vi "MovementDirections.vi"(9 "Key input":T1, 10 "Level input":u32[][](array[colorbox]), 11 "Location input":cluster{"Y":i32, "X":i32}[](array[cluster])=[{"Y"=12, "X"=8}, {"Y"=12, "X"=7}, {"Y"=12, "X"=6}, {"Y"=12, "X"=5}]) -> (1 "Key output":T1, 2 "Level output":u32[][](array[colorbox]), 3 "Location output":cluster{"Y":i32, "X":i32}[](array[cluster])=[{"Y"=12, "X"=8}, {"Y"=12, "X"=7}, {"Y"=12, "X"=6}, {"Y"=12, "X"=5}])   [LabVIEW 2021]
uses:
  TypeDef/KeyDown.ctl
  GlobalVariables/Board_Colors.vi
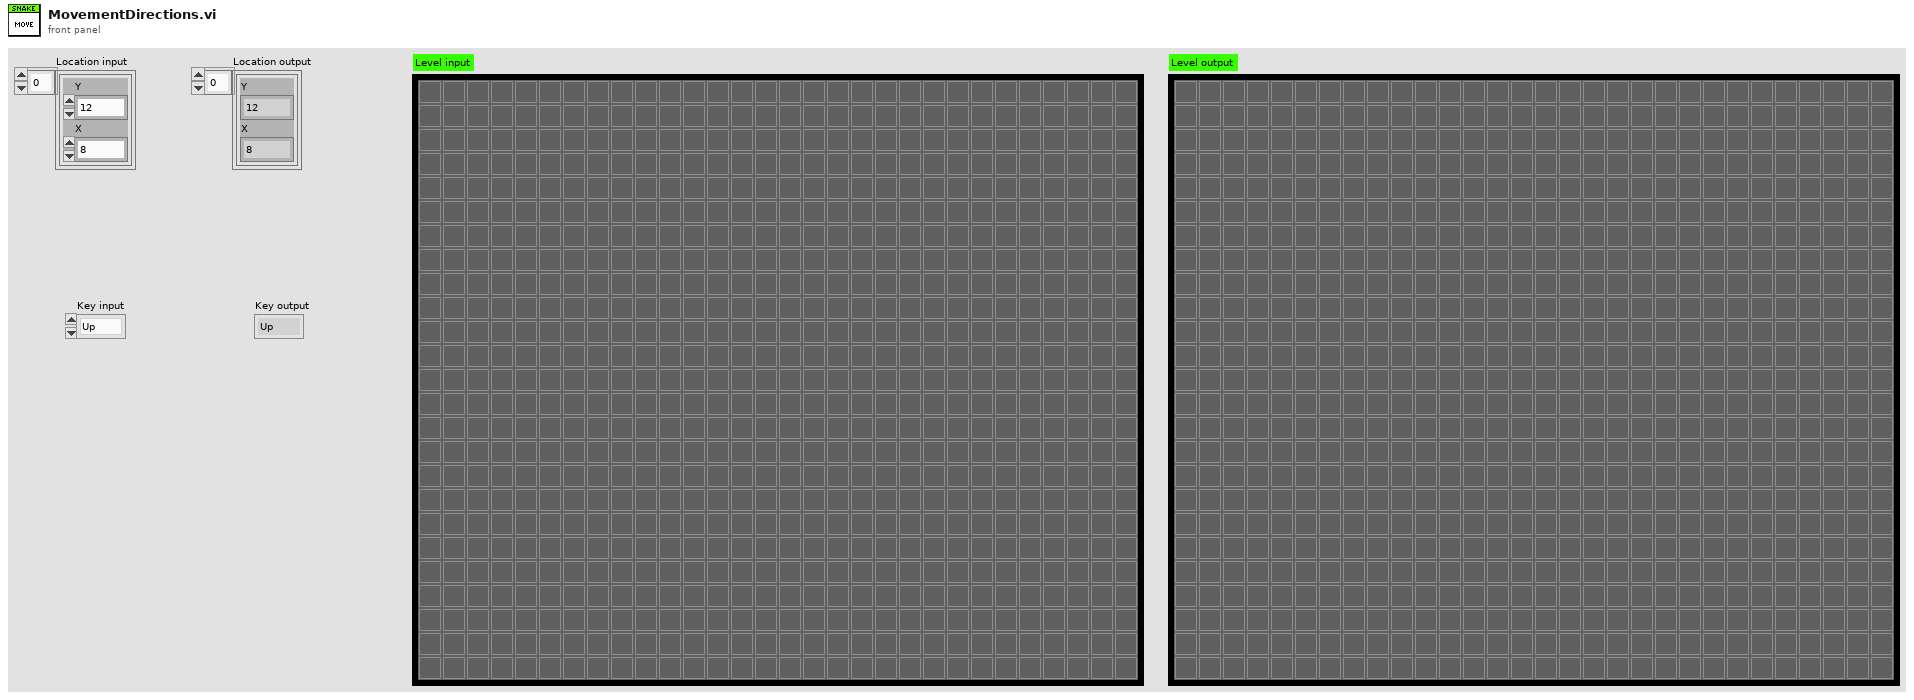
[diagram p1: front panel]
types:
  T1 = typedef "KeyDown.ctl" = enum16{"Up", "Down", "Left", "Right"}
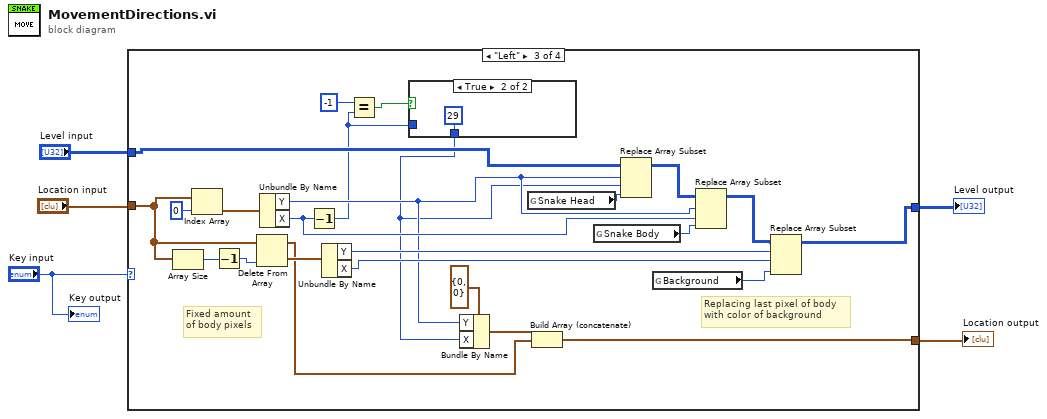
[diagram p0: block diagram]
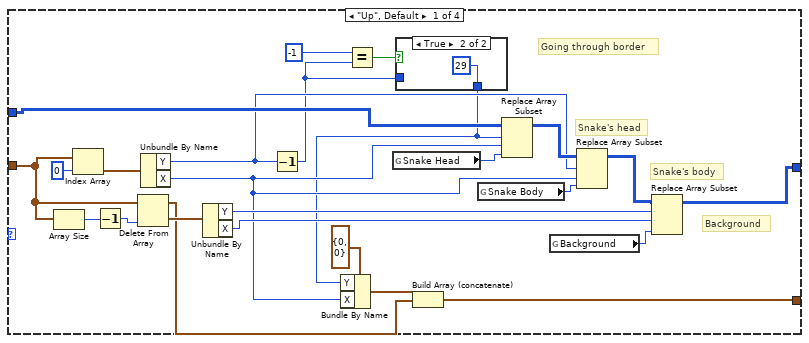
[diagram p2: hidden frame]
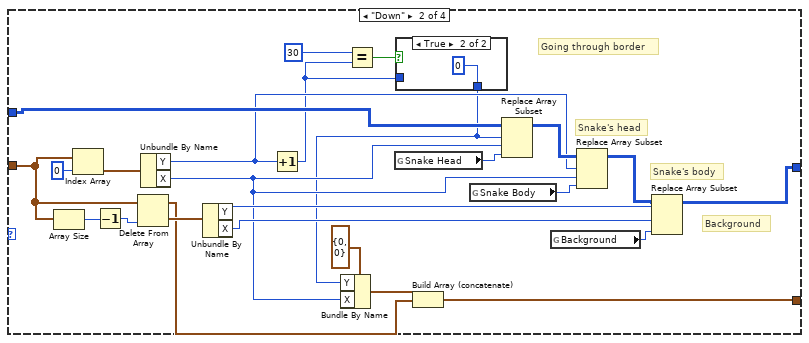
[diagram p4: hidden frame]
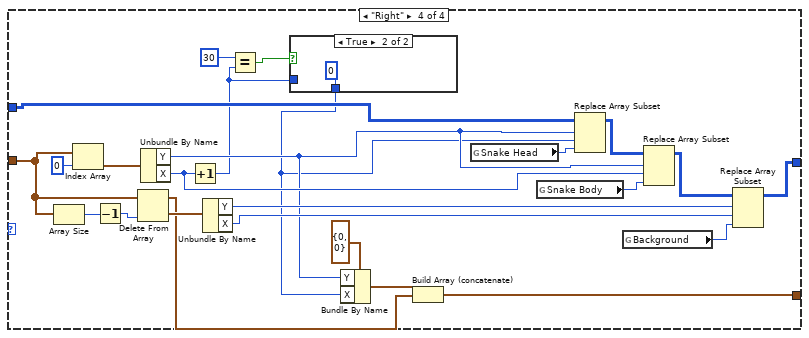
[diagram p7: hidden frame]
diagram:
  n1 = case shown="\"Left\"" "Key input" {
    tunnel: "Level input" -> [w27 w54 w81 w108]
    tunnel: [w22 w49 w75 w102] -> w3
    tunnel: "Location input" -> [w19 w46 w71 w98]
    tunnel: [w15 w42 w67 w94] -> w1
    frame "Up", Default {
      # "Background"
      # "Snake's body"
      # "Snake's head"
      # "Going through border"
      n2 = Array Size(array=w19) -> (size(s)=w28:i32)
      n3 = Index Array(array=w19, index=0) -> (element=w29:cluster{"Y":i32, "X":i32})
      n4 = Decrement(x=w28) -> (x-1=w18:i32)
      n5 = Delete From Array(array=w19, index=w18) -> (deleted portion=w17:cluster{"Y":i32, "X":i32}, array with subset deleted=w16:cluster{"Y":i32, "X":i32}[])  [unwired: 1 in]
      n6 = Unbundle By Name(w29) -> ("Y"=w13:i32, "X"=w14:i32)
      n7 = Unbundle By Name(w17) -> ("Y"=w24:i32, "X"=w23:i32)
      n8 = Decrement(x=w13) -> (x-1=w10:i32)
      n9 = Equal?(x=-1, y=w10) -> (x = y?=w12:bool)
      n10 = global read "Board_Colors.vi" "Snake Head"() -> (w6:u32)
      n11 = case shown="True" w12 {
        tunnel: [w31 29] -> w9
        tunnel: w10 -> [w31 _]
        frame False {
        }
        frame True {
        }
      }
      n12 = Bundle By Name(cluster=cluster{"Y":i32, "X":i32} {"Y"=0, "X"=0} ("input cluster"), "Y"=w9, "X"=w14) -> (w20:cluster{"Y":i32, "X":i32})
      n13 = Build Array (concatenate)(w20, w16) -> (w15:cluster{"Y":i32, "X":i32}[])
      n14 = global read "Board_Colors.vi" "Snake Body"() -> (w7:u32)
      n15 = Replace Array Subset(array=w27, new element=w6, index (row)=w9, index (col)=w14) -> (w26:u32[][])
      n16 = global read "Board_Colors.vi" "Background"() -> (w8:u32)
      n17 = Replace Array Subset(array=w26, new element=w7, index (row)=w13, index (col)=w14) -> (w25:u32[][])
      n18 = Replace Array Subset(array=w25, new element=w8, index (row)=w24, index (col)=w23) -> (w22:u32[][])
    }
    frame "Down" {
      # "Background"
      # "Snake's body"
      # "Snake's head"
      # "Going through border"
      n19 = Array Size(array=w46) -> (size(s)=w55:i32)
      n20 = Index Array(array=w46, index=0) -> (element=w56:cluster{"Y":i32, "X":i32})
      n21 = Decrement(x=w55) -> (x-1=w45:i32)
      n22 = Delete From Array(array=w46, index=w45) -> (deleted portion=w44:cluster{"Y":i32, "X":i32}, array with subset deleted=w43:cluster{"Y":i32, "X":i32}[])  [unwired: 1 in]
      n23 = Unbundle By Name(w56) -> ("Y"=w40:i32, "X"=w41:i32)
      n24 = Unbundle By Name(w44) -> ("Y"=w51:i32, "X"=w50:i32)
      n25 = Increment(x=w40) -> (x+1=w37:i32)
      n26 = Equal?(x=30, y=w37) -> (x = y?=w39:bool)
      n27 = global read "Board_Colors.vi" "Snake Head"() -> (w33:u32)
      n28 = case shown="True" w39 {
        tunnel: [w58 0] -> w36
        tunnel: w37 -> [w58 _]
        frame False {
        }
        frame True {
        }
      }
      n29 = Bundle By Name(cluster=cluster{"Y":i32, "X":i32} {"Y"=0, "X"=0} ("input cluster"), "Y"=w36, "X"=w41) -> (w47:cluster{"Y":i32, "X":i32})
      n30 = Build Array (concatenate)(w47, w43) -> (w42:cluster{"Y":i32, "X":i32}[])
      n31 = global read "Board_Colors.vi" "Snake Body"() -> (w34:u32)
      n32 = Replace Array Subset(array=w54, new element=w33, index (row)=w36, index (col)=w41) -> (w53:u32[][])
      n33 = global read "Board_Colors.vi" "Background"() -> (w35:u32)
      n34 = Replace Array Subset(array=w53, new element=w34, index (row)=w40, index (col)=w41) -> (w52:u32[][])
      n35 = Replace Array Subset(array=w52, new element=w35, index (row)=w51, index (col)=w50) -> (w49:u32[][])
    }
    frame "Left" {
      # "Fixed amount\nof body pixels"
      # "Replacing last pixel of body\nwith color of background"
      n36 = Array Size(array=w71) -> (size(s)=w82:i32)
      n37 = Index Array(array=w71, index=0) -> (element=w83:cluster{"Y":i32, "X":i32})
      n38 = Decrement(x=w82) -> (x-1=w70:i32)
      n39 = Delete From Array(array=w71, index=w70) -> (deleted portion=w69:cluster{"Y":i32, "X":i32}, array with subset deleted=w68:cluster{"Y":i32, "X":i32}[])  [unwired: 1 in]
      n40 = Unbundle By Name(w83) -> ("Y"=w74:i32, "X"=w76:i32)
      n41 = Decrement(x=w76) -> (x-1=w63:i32)
      n42 = Unbundle By Name(w69) -> ("Y"=w78:i32, "X"=w77:i32)
      n43 = Equal?(x=-1, y=w63) -> (x = y?=w65:bool)
      n44 = case shown="True" w65 {
        tunnel: [w85 29] -> w64
        tunnel: w63 -> [w85 _]
        frame False {
        }
        frame True {
        }
      }
      n45 = Bundle By Name(cluster=cluster{"Y":i32, "X":i32} {"Y"=0, "X"=0} ("input cluster"), "Y"=w74, "X"=w64) -> (w72:cluster{"Y":i32, "X":i32})
      n46 = global read "Board_Colors.vi" "Snake Head"() -> (w61:u32)
      n47 = Build Array (concatenate)(w72, w68) -> (w67:cluster{"Y":i32, "X":i32}[])
      n48 = global read "Board_Colors.vi" "Snake Body"() -> (w60:u32)
      n49 = Replace Array Subset(array=w81, new element=w61, index (row)=w74, index (col)=w64) -> (w80:u32[][])
      n50 = global read "Board_Colors.vi" "Background"() -> (w62:u32)
      n51 = Replace Array Subset(array=w80, new element=w60, index (row)=w74, index (col)=w76) -> (w79:u32[][])
      n52 = Replace Array Subset(array=w79, new element=w62, index (row)=w78, index (col)=w77) -> (w75:u32[][])
    }
    frame "Right" {
      n53 = Array Size(array=w98) -> (size(s)=w109:i32)
      n54 = Index Array(array=w98, index=0) -> (element=w110:cluster{"Y":i32, "X":i32})
      n55 = Decrement(x=w109) -> (x-1=w97:i32)
      n56 = Delete From Array(array=w98, index=w97) -> (deleted portion=w96:cluster{"Y":i32, "X":i32}, array with subset deleted=w95:cluster{"Y":i32, "X":i32}[])  [unwired: 1 in]
      n57 = Unbundle By Name(w110) -> ("Y"=w101:i32, "X"=w103:i32)
      n58 = Increment(x=w103) -> (x+1=w90:i32)
      n59 = Unbundle By Name(w96) -> ("Y"=w105:i32, "X"=w104:i32)
      n60 = Equal?(x=30, y=w90) -> (x = y?=w92:bool)
      n61 = case shown="True" w92 {
        tunnel: [w112 0] -> w91
        tunnel: w90 -> [w112 _]
        frame False {
        }
        frame True {
        }
      }
      n62 = Bundle By Name(cluster=cluster{"Y":i32, "X":i32} {"Y"=0, "X"=0} ("input cluster"), "Y"=w101, "X"=w91) -> (w99:cluster{"Y":i32, "X":i32})
      n63 = Build Array (concatenate)(w99, w95) -> (w94:cluster{"Y":i32, "X":i32}[])
      n64 = global read "Board_Colors.vi" "Snake Head"() -> (w87:u32)
      n65 = global read "Board_Colors.vi" "Snake Body"() -> (w88:u32)
      n66 = Replace Array Subset(array=w108, new element=w87, index (row)=w101, index (col)=w91) -> (w107:u32[][])
      n67 = global read "Board_Colors.vi" "Background"() -> (w89:u32)
      n68 = Replace Array Subset(array=w107, new element=w88, index (row)=w101, index (col)=w103) -> (w106:u32[][])
      n69 = Replace Array Subset(array=w106, new element=w89, index (row)=w105, index (col)=w104) -> (w102:u32[][])
    }
  }
  "Level output" <- w3
  "Location output" <- w1
  "Key output" <- "Key input"
